vi "IT6726Control.vi"(9 "输入":dbl, 10 "VISA resource name":refnum<visa-resource-name> caption="VISA资源名称", 11 "Sequence Context In":refnum<k7>) -> (0 "error out":errorcluster, 1 "输出":dbl, 3 "Report Text":string)   [LabVIEW 2013]
uses:
  <vilib>/Instr/_visa.llb/VISA Configure Serial Port (Instr).vi
panel:
  in  "功能":T1(ring)
  in  "error in (no error)":errorcluster caption="错误输入（无错误）"
  # "IT6726 CONTROL"
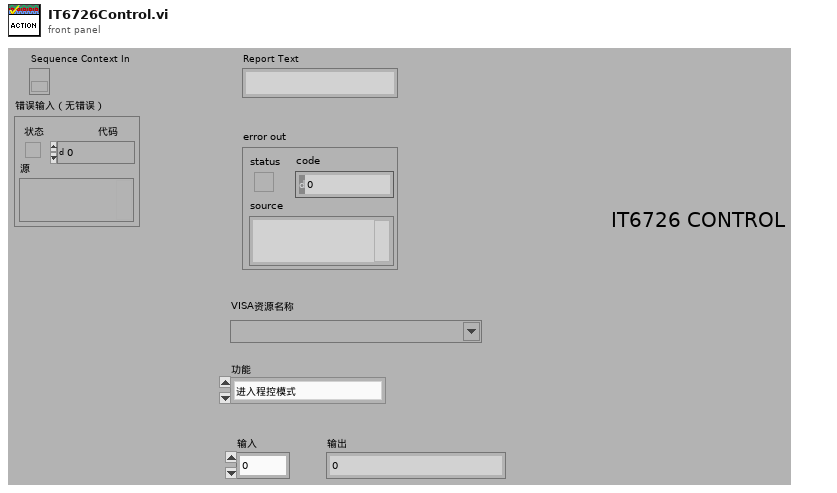
[diagram p1: front panel]
types:
  T1 = enum16{"进入程控模式", "输出ON", "输出OFF", "设置电压", "设置电流", "读取电压", "读取电流"}
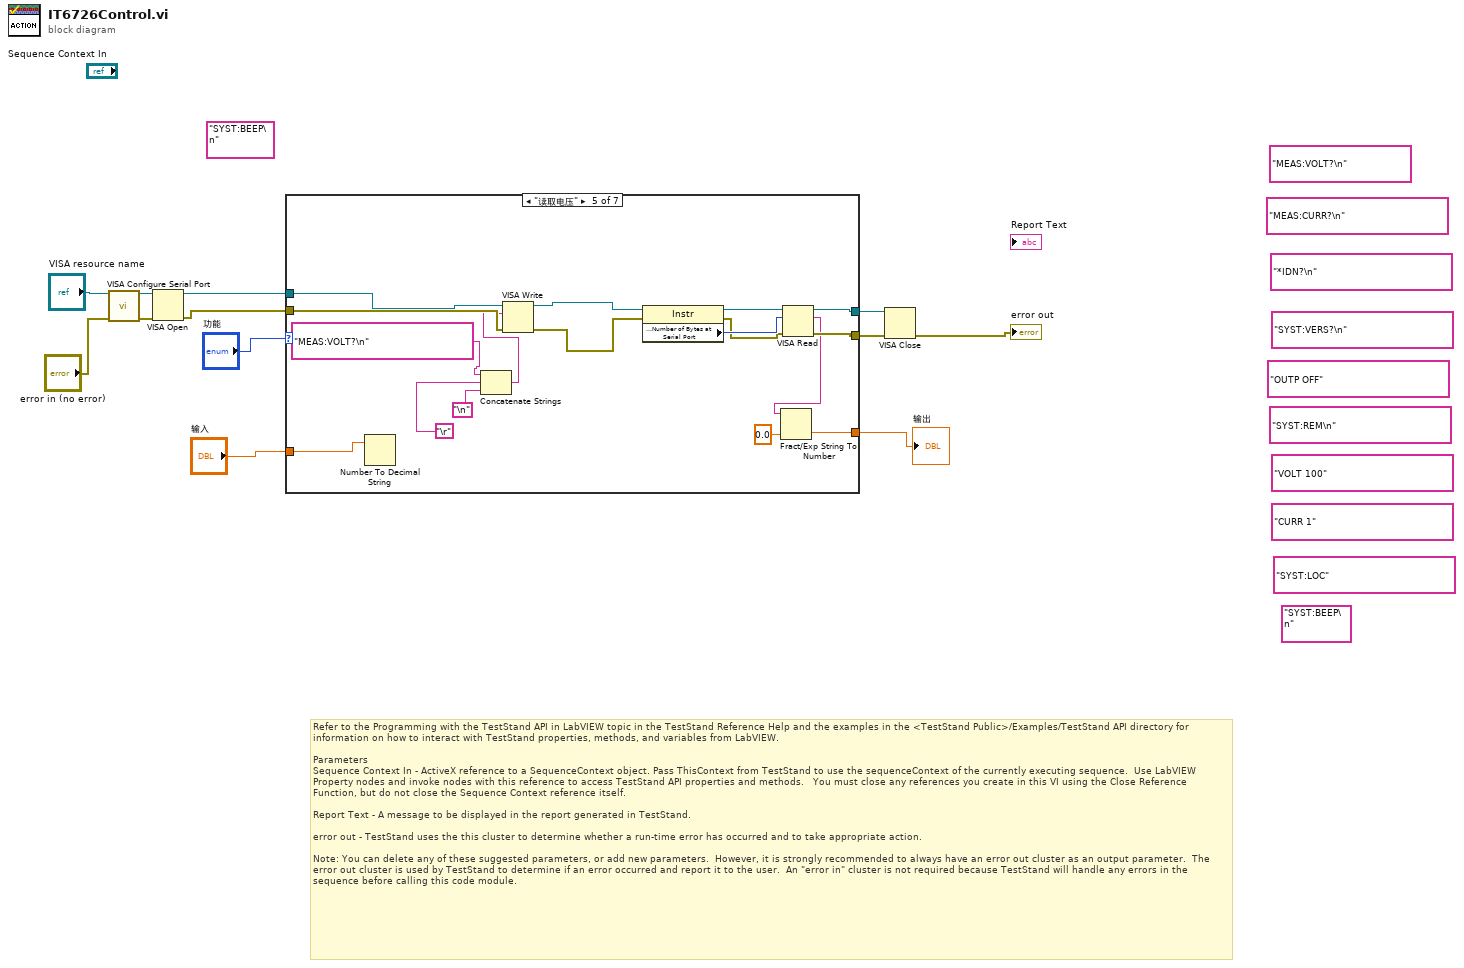
[diagram p0: block diagram]
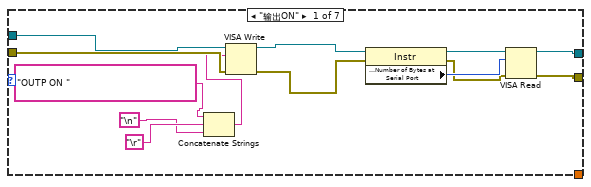
[diagram p2: hidden frame]
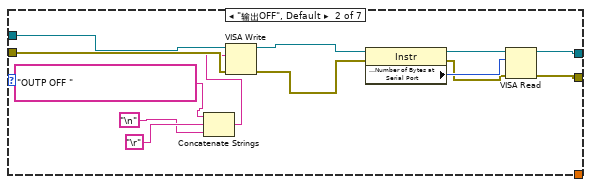
[diagram p3: hidden frame]
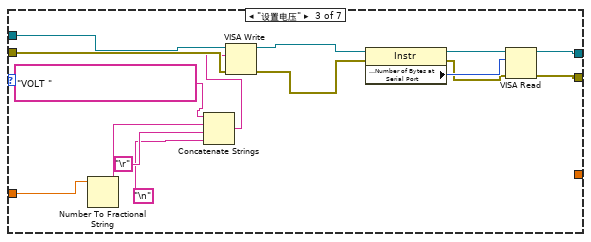
[diagram p4: hidden frame]
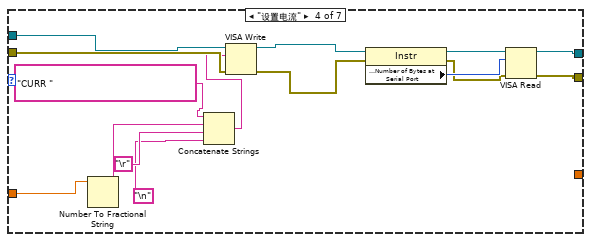
[diagram p5: hidden frame]
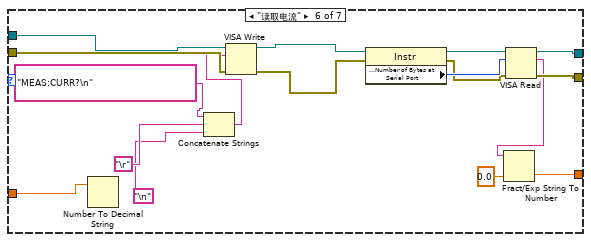
[diagram p6: hidden frame]
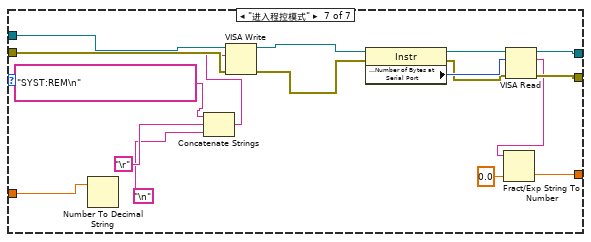
[diagram p7: hidden frame]
diagram:
  (unwired) "SYST:LOC" ("写入缓冲区")
  (unwired) "CURR 1" ("写入缓冲区")
  (unwired) "VOLT 100" ("写入缓冲区")
  (unwired) "OUTP OFF" ("写入缓冲区")
  (unwired) "SYST:REM\n" ("写入缓冲区")
  (unwired) "SYST:VERS?\n" ("写入缓冲区")
  (unwired) "*IDN?\n" ("写入缓冲区")
  (unwired) "MEAS:CURR?\n" ("写入缓冲区")
  (unwired) "MEAS:VOLT?\n" ("写入缓冲区")
  (unwired) "SYST:BEEP\n" ("写入缓冲区")
  (unwired) "SYST:BEEP\n" ("写入缓冲区")
  # "Refer to the Programming with the TestStand API in LabVIEW topic in the TestStand Reference Help and the examples in the <TestStand Public>/Examples/TestStand API directory for information on how to interact with TestStand properties, methods, and variables from LabVIEW.\n\nParameters\nSequence Context In - ActiveX reference to a SequenceContext object. Pass ThisContext from TestStand to use the sequenceContext of the currently executing sequence.  Use LabVIEW Property nodes and invoke nodes with this reference to access TestStand API properties and methods.   You must close any references you create in this VI using the Close Reference Function, but do not close the Sequence Context reference itself.\n\nReport Text - A message to be displayed in the report generated in TestStand. \n\nerror out - TestStand uses the this cluster to determine whether a run-time error has occurred and to take appropriate action.  \n\nNote: You can delete any of these suggested parameters, or add new parameters.  However, it is strongly recommended to always have an error out cluster as an output parameter.  The error out cluster is used by TestStand to determine if an error occurred and report it to the user.  An \"error in\" cluster is not required because TestStand will handle any errors in the sequence before calling this code module."
  n1 = call-poly "VISA Configure Serial Port"("VISA resource name"="VISA resource name", "error in (no error)"="error in (no error)") -> ("VISA resource name out"=w10:refnum<visa-resource-name>, "error out"=w11:errorcluster)  [unwired: 12 in]
  n2 = VISA Open(error in (no error)=w11, VISA resource name=w10) -> (VISA resource name=w9:refnum<visa-resource-name>, error out=w8:errorcluster)  [unwired: 3 in]
  n3 = case shown="\"读取电压\"" "功能" {
    tunnel: w9 -> [w25 w38 w53 w68 w85 w102 w119]
    tunnel: w8 -> [w24 w37 w52 w67 w84 w101 w118]
    tunnel: [w16 w29 w44 w59 w76 w93 w110] -> w6
    tunnel: [w15 w28 w43 w58 w75 w92 w109] -> w5
    tunnel: "输入" -> [_ _ w39 w54 w72 w89 w106]
    tunnel: [_ _ _ _ w69 w86 w103] -> w1
    frame "输出ON" {
      n4 = Concatenate Strings("OUTP ON " ("写入缓冲区"), "\r", "\n") -> (w19:string)
      n5 = VISA Write(VISA resource name=w25, write buffer=w19, error in (no error)=w24) -> (VISA resource name out=w23:refnum<visa-resource-name>, error out=w13:errorcluster)  [unwired: 1 out]
      n6 = property class="Instr"(reference=w23, error in=w13) -> (reference out=w22:refnum<visa-resource-name>, error out=w14:errorcluster, "Serial Settings:Number of Bytes at Serial Port"=w21:u32)
      n7 = VISA Read(VISA resource name=w22, byte count=w21, error in (no error)=w14) -> (VISA resource name out=w16:refnum<visa-resource-name>, error out=w15:errorcluster)  [unwired: 2 out]
    }
    frame "输出OFF", Default {
      n8 = Concatenate Strings("OUTP OFF " ("写入缓冲区"), "\r", "\n") -> (w32:string)
      n9 = VISA Write(VISA resource name=w38, write buffer=w32, error in (no error)=w37) -> (VISA resource name out=w36:refnum<visa-resource-name>, error out=w26:errorcluster)  [unwired: 1 out]
      n10 = property class="Instr"(reference=w36, error in=w26) -> (reference out=w35:refnum<visa-resource-name>, error out=w27:errorcluster, "Serial Settings:Number of Bytes at Serial Port"=w34:u32)
      n11 = VISA Read(VISA resource name=w35, byte count=w34, error in (no error)=w27) -> (VISA resource name out=w29:refnum<visa-resource-name>, error out=w28:errorcluster)  [unwired: 2 out]
    }
    frame "设置电压" {
      n12 = Number To Fractional String(number=w39) -> (F-format string=w40:string)  [unwired: 3 in]
      n13 = Concatenate Strings("VOLT " ("写入缓冲区"), w40, "\r", "\n") -> (w47:string)
      n14 = VISA Write(VISA resource name=w53, write buffer=w47, error in (no error)=w52) -> (VISA resource name out=w51:refnum<visa-resource-name>, error out=w41:errorcluster)  [unwired: 1 out]
      n15 = property class="Instr"(reference=w51, error in=w41) -> (reference out=w50:refnum<visa-resource-name>, error out=w42:errorcluster, "Serial Settings:Number of Bytes at Serial Port"=w49:u32)
      n16 = VISA Read(VISA resource name=w50, byte count=w49, error in (no error)=w42) -> (VISA resource name out=w44:refnum<visa-resource-name>, error out=w43:errorcluster)  [unwired: 2 out]
    }
    frame "设置电流" {
      n17 = Number To Fractional String(number=w54) -> (F-format string=w55:string)  [unwired: 3 in]
      n18 = Concatenate Strings("CURR " ("写入缓冲区"), w55, "\r", "\n") -> (w62:string)
      n19 = VISA Write(VISA resource name=w68, write buffer=w62, error in (no error)=w67) -> (VISA resource name out=w66:refnum<visa-resource-name>, error out=w56:errorcluster)  [unwired: 1 out]
      n20 = property class="Instr"(reference=w66, error in=w56) -> (reference out=w65:refnum<visa-resource-name>, error out=w57:errorcluster, "Serial Settings:Number of Bytes at Serial Port"=w64:u32)
      n21 = VISA Read(VISA resource name=w65, byte count=w64, error in (no error)=w57) -> (VISA resource name out=w59:refnum<visa-resource-name>, error out=w58:errorcluster)  [unwired: 2 out]
    }
    frame "读取电压" {
      n22 = Number To Decimal String(number=w72) -> ()  [unwired: 1 in, 1 out]
      n23 = Concatenate Strings("MEAS:VOLT?\n" ("写入缓冲区"), "\r", "\n") -> (w79:string)
      n24 = VISA Write(VISA resource name=w85, write buffer=w79, error in (no error)=w84) -> (VISA resource name out=w83:refnum<visa-resource-name>, error out=w73:errorcluster)  [unwired: 1 out]
      n25 = property class="Instr"(reference=w83, error in=w73) -> (reference out=w82:refnum<visa-resource-name>, error out=w74:errorcluster, "Serial Settings:Number of Bytes at Serial Port"=w81:u32)
      n26 = VISA Read(VISA resource name=w82, byte count=w81, error in (no error)=w74) -> (VISA resource name out=w76:refnum<visa-resource-name>, read buffer=w71:string, error out=w75:errorcluster)  [unwired: 1 out]
      n27 = Fract/Exp String To Number(string=w71, default (0 dbl)=0.0 ("默认(0 I32)")) -> (number=w69:dbl)  [unwired: 2 in, 1 out]
    }
    frame "读取电流" {
      n28 = Number To Decimal String(number=w89) -> ()  [unwired: 1 in, 1 out]
      n29 = Concatenate Strings("MEAS:CURR?\n" ("写入缓冲区"), "\r", "\n") -> (w96:string)
      n30 = VISA Write(VISA resource name=w102, write buffer=w96, error in (no error)=w101) -> (VISA resource name out=w100:refnum<visa-resource-name>, error out=w90:errorcluster)  [unwired: 1 out]
      n31 = property class="Instr"(reference=w100, error in=w90) -> (reference out=w99:refnum<visa-resource-name>, error out=w91:errorcluster, "Serial Settings:Number of Bytes at Serial Port"=w98:u32)
      n32 = VISA Read(VISA resource name=w99, byte count=w98, error in (no error)=w91) -> (VISA resource name out=w93:refnum<visa-resource-name>, read buffer=w88:string, error out=w92:errorcluster)  [unwired: 1 out]
      n33 = Fract/Exp String To Number(string=w88, default (0 dbl)=0.0 ("默认(0 I32)")) -> (number=w86:dbl)  [unwired: 2 in, 1 out]
    }
    frame "进入程控模式" {
      n34 = Number To Decimal String(number=w106) -> ()  [unwired: 1 in, 1 out]
      n35 = Concatenate Strings("SYST:REM\n" ("写入缓冲区"), "\r", "\n") -> (w113:string)
      n36 = VISA Write(VISA resource name=w119, write buffer=w113, error in (no error)=w118) -> (VISA resource name out=w117:refnum<visa-resource-name>, error out=w107:errorcluster)  [unwired: 1 out]
      n37 = property class="Instr"(reference=w117, error in=w107) -> (reference out=w116:refnum<visa-resource-name>, error out=w108:errorcluster, "Serial Settings:Number of Bytes at Serial Port"=w115:u32)
      n38 = VISA Read(VISA resource name=w116, byte count=w115, error in (no error)=w108) -> (VISA resource name out=w110:refnum<visa-resource-name>, read buffer=w105:string, error out=w109:errorcluster)  [unwired: 1 out]
      n39 = Fract/Exp String To Number(string=w105, default (0 dbl)=0.0 ("默认(0 I32)")) -> (number=w103:dbl)  [unwired: 2 in, 1 out]
    }
  }
  "输出" <- w1
  n40 = VISA Close(VISA resource name=w6, error in (no error)=w5) -> (error out=→"error out":errorcluster)
